vi "IMAQ FPGA Data Valid Bool Array to Int.vi"(11 "DV In":bool[](array[boolean])=[FALSE, FALSE, FALSE, FALSE, FALSE, FALSE, FALSE, FALSE]) -> (3 "Sum DV Out":u8)   [LabVIEW 2017, in "NI_VDM_FPGA_Basics.lvlib"]
uses:
  <vilib>/visionFPGA/NI_VDM_FPGA_Basics.lvlib
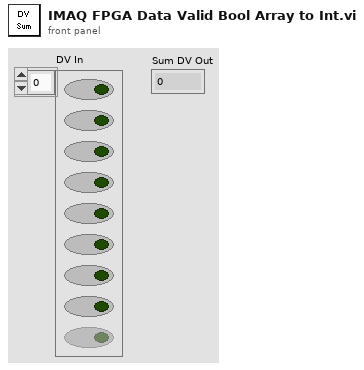
[diagram p1: front panel]
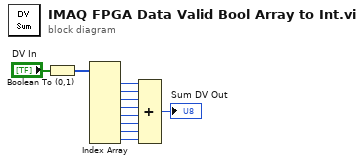
[diagram p0: block diagram]
diagram:
  n1 = Boolean To (0,1)(Boolean="DV In") -> (0, 1=w10:i16[])
  n2 = Index Array(array=w10) -> (element #1=w9:i16, element #2=w8:i16, element #3=w2:i16, element #4=w3:i16, element #5=w4:i16, element #6=w5:i16, element #7=w6:i16, element #8=w7:i16)  [unwired: 8 in]
  n3 = Compound Arithmetic op=ADD(w9, w8, w2, w3, w4, w5, w6, w7) -> (→"Sum DV Out":i16)
